vi "Get Component Type.vi"(8 "error in (no error)":errorcluster, 11 "SMOFacade in":refnum<class "SMOFacade.lvclass">) -> (0 "error out":errorcluster, 2 "Class Name":string, 3 "SMOFacade out":refnum<class "SMOFacade.lvclass">)   [LabVIEW 2013, in "SMOFacade.lvclass"]
uses:
  SMOFacade.lvclass
  SMOFacade.lvclass/SMOFacade.ctl
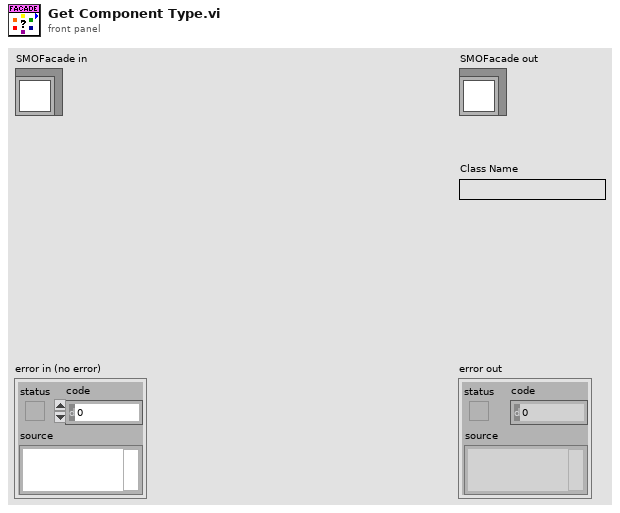
[diagram p1: front panel]
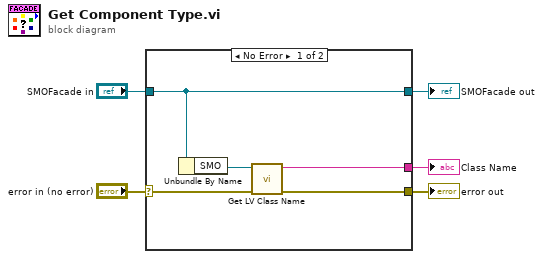
[diagram p0: block diagram]
diagram:
  n1 = case shown="No Error" "error in (no error)" {
    selector: "error in (no error)" -> [w8 w12]
    tunnel: [w7 w12] -> w4
    tunnel: [w10 w11] -> w2
    tunnel: "SMOFacade in" -> [w10 w11]
    tunnel: [w6 _] -> w1
    frame No Error {
      n2 = Unbundle By Name(w10) -> ("SMO"=w9:refnum<class "SMO.lvclass">)
      n3 = call <vilib>:"Get LV Class Name.vi"("error in (no error)"=w8, "object"=w9) -> ("error out"=w7:errorcluster, "class name"=w6:string)  [unwired: 8 in]
    }
    frame Error {
    }
  }
  "error out" <- w4
  "SMOFacade out" <- w2
  "Class Name" <- w1
